vi "4Pi 4Pi Modes - DM AE.vi"(0 "DM Handles":T1(array[cluster]), 1 "Action":T2, 7 "Flats":dbl[](array[numeric]), 11 "Control Matrix":dbl[][](array[numeric]), 12 "No hardware":bool=TRUE) -> (4 "DM Handles Out":T1(array[cluster]), 8 "Flats Out":dbl[](array[numeric]), 14 "No hardware Out":bool, 15 "Control Matrix Out":dbl[][](array[numeric]))   [LabVIEW 2016]
uses:
  4Pi 4Pi Modes - Controls/4Pi 4Pi Modes - Standard Action.ctl
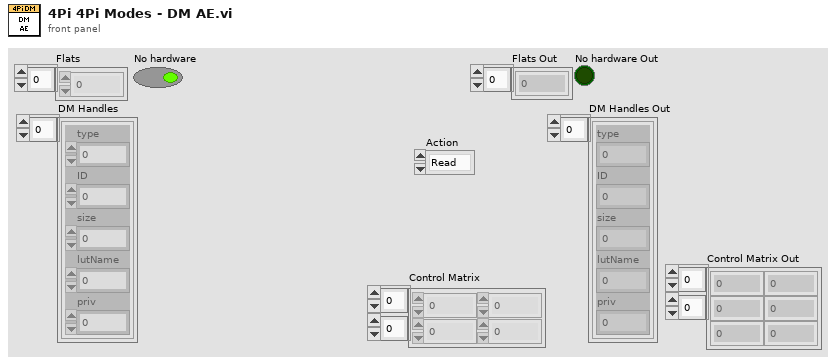
[diagram p1: front panel]
types:
  T1 = cluster{"type":i16, "ID":i16, "size":i32, "lutName":u64, "priv":u64}[]
  T2 = typedef "4Pi 4Pi Modes - Standard Action.ctl" = enum16{"Read", "Write"}
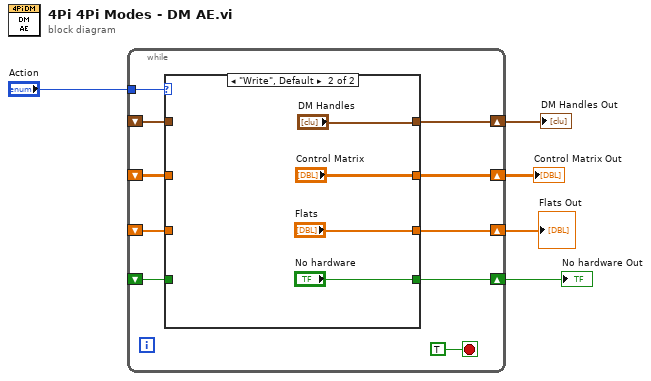
[diagram p0: block diagram]
diagram:
  n1 = while {
    tunnel: "Action" -> [w14]
    shift-right: [w10] -> w3
    shift-left: _ -> [w13]
    shift-right: [w12] -> w4
    shift-left: _ -> [w11]
    shift-right: [w9] -> w2
    shift-left: _ -> [w8]
    shift-right: [w7] -> w1
    shift-left: _ -> [w6]
    stop <- TRUE stop-if-true
    n2 = case shown="\"Write\", Default" w14 {
      tunnel: w13 -> [w18 _]
      tunnel: [w19 "Control Matrix"] -> w12
      tunnel: w11 -> [w19 _]
      tunnel: [w18 "Flats"] -> w10
      tunnel: [w17 "DM Handles"] -> w9
      tunnel: w8 -> [w17 _]
      tunnel: [w16 "No hardware"] -> w7
      tunnel: w6 -> [w16 _]
      frame "Read" {
      }
      frame "Write", Default {
      }
    }
  }
  "Control Matrix Out" <- w4
  "Flats Out" <- w3
  "DM Handles Out" <- w2
  "No hardware Out" <- w1
